vi "Car Wash.vi"() -> ()   [LabVIEW 2018]
uses:
  Controls/Car Wash Indicators.ctl
  Controls/Wash Options.ctl
  Controls/Timer Parameters.ctl
  Controls/FGV Timer Control.ctl
  Controls/UI Data Car Wash.ctl
  Controls/Wash Option Parameters.ctl
  support/Message Queue/Enqueue Message (Single).vi
  <vilib>/Utility/error.llb/Error Cluster From Error Code.vi
  <vilib>/ErrorRing/Error Ring.xnode
  support/Message Queue/Message Queue.lvlib
  support/User Event - Stop/User Event - Stop.lvlib
panel:
  in  "Start":bool
  out "Elapsed Time":dbl format="%0.2f"
  in  "stop":bool
  out "Wash Entry":bool
  in  "Wash Options":T1
  in  "Car Position Slider":u8(slide) max=3 scale=0.0..4.0
  out "Car Wash Indicators":T2
  # "Entry Console"
  # "Car Wash Display"
  # "Car Position Simulation"
  # "Pre-Soak\nH-P Wash\nL-P Wax\nSpot Free Rinse"
  # "Underbody Wash\nBug Remover"
  # "Tire Shine\nAir Dry"
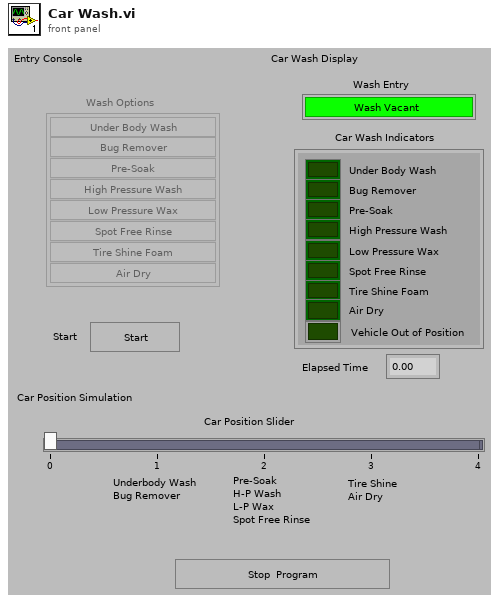
[diagram p1: front panel]
types:
  T1 = typedef "Wash Options.ctl" = cluster{"Underbody Wash":bool, "Bug Remover":bool, "Pre-Soak":bool, "High Pressure Wash":bool, "Low Pressure Wax":bool, "Spot Free Rinse":bool, "Tire Shine Foam":bool, "Air Dry":bool}
  T2 = typedef "Car Wash Indicators.ctl" = cluster{"Under Body Wash":bool, "Bug Remover":bool, "Pre-Soak":bool, "High Pressure Wash":bool, "Low Pressure Wax":bool, "Spot Free Rinse":bool, "Tire Shine Foam":bool, "Air Dry":bool, "Vehicle Out of Position":bool}
  T3 = typedef "UI Data Car Wash.ctl" = cluster{"Underbody Wash Ref":refnum<vi>, "Bug Remover Ref":refnum<vi>, "Pre-Soak Ref":refnum<vi>, "High Pressure Ref":refnum<vi>, "Low Pressure Ref":refnum<vi>, "Spot Free Rinse Ref":refnum<vi>, "Tire Shine Foam Ref":refnum<vi>, "Air Dry Ref":refnum<vi>}
  T4 = typedef "Timer Parameters.ctl" = cluster{"Time Target":dbl, "Timer Mode":T5}
  T5 = typedef "FGV Timer Control.ctl" = enum16{"Start Time", "Read Time", "Pause", "Resume"}
  T6 = typedef "Message Queue.lvlib/All Message Queues.ctl" = cluster{"UI":refnum<queue>}
  T7 = enum8{"Enabled", "Disabled", "Disabled and Grayed Out"}
  T8 = typedef "Wash Option Parameters.ctl" = cluster{"Wash Option":string, "Time":i32, "Station":i32}
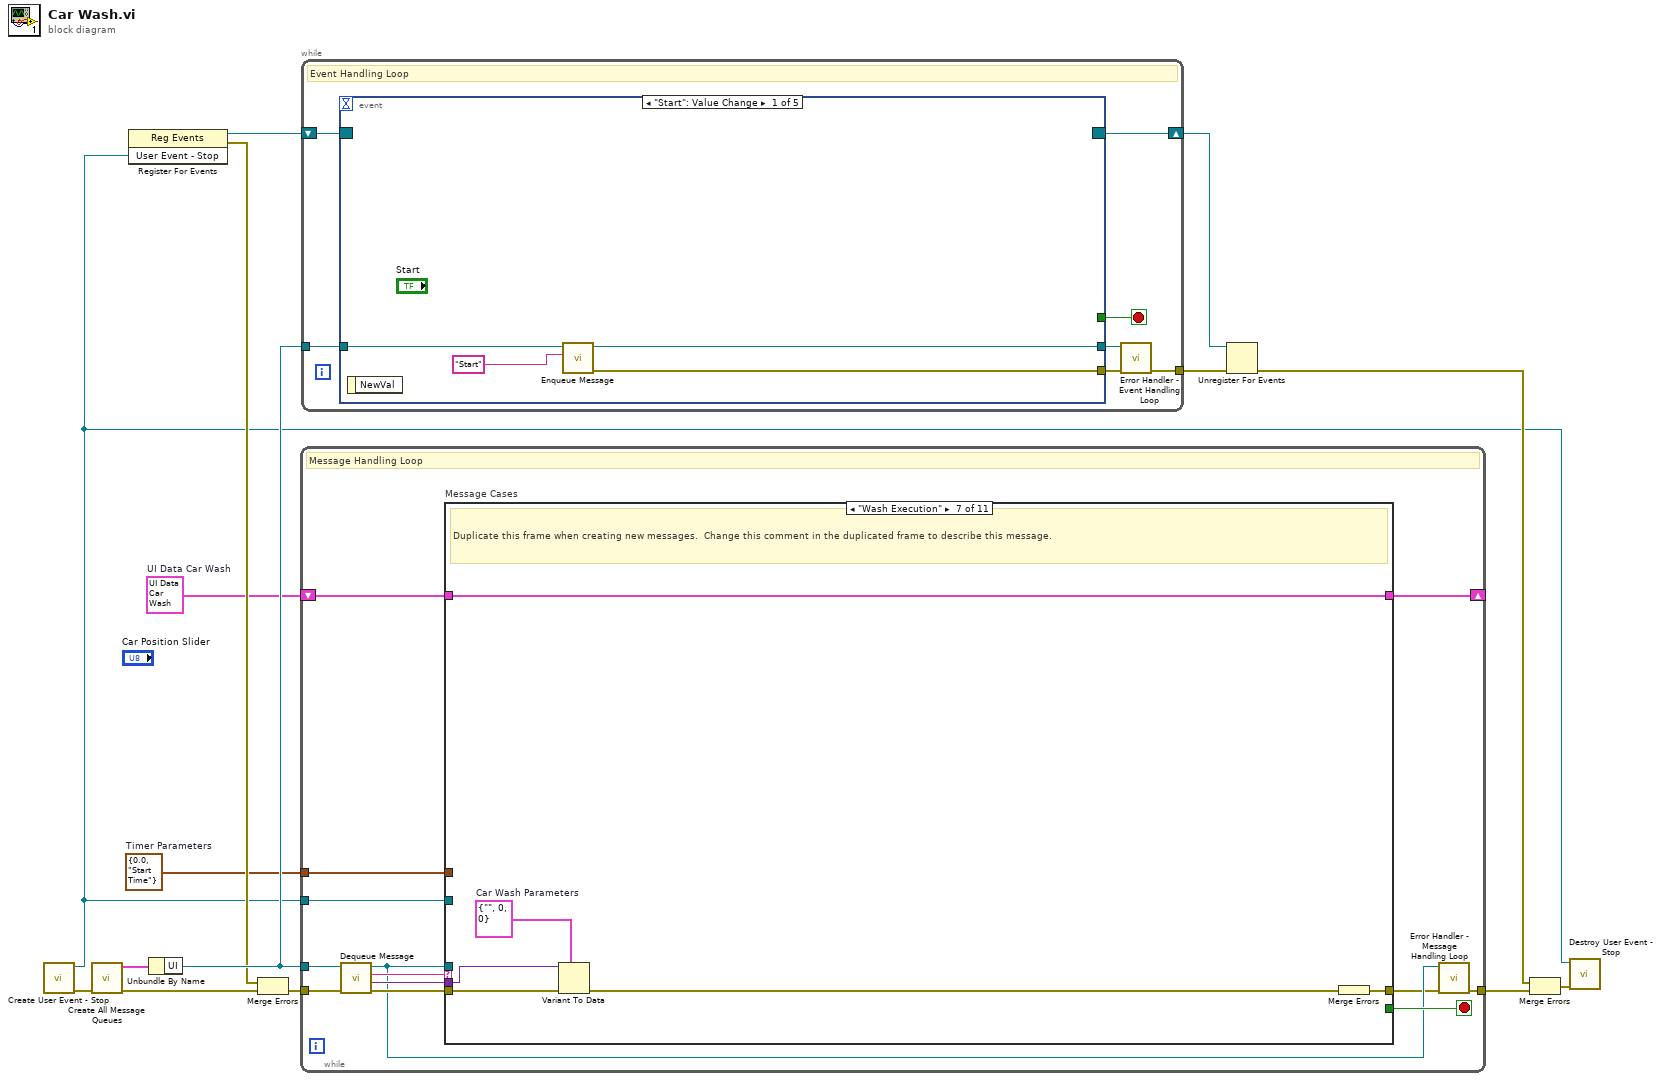
[diagram p0: block diagram]
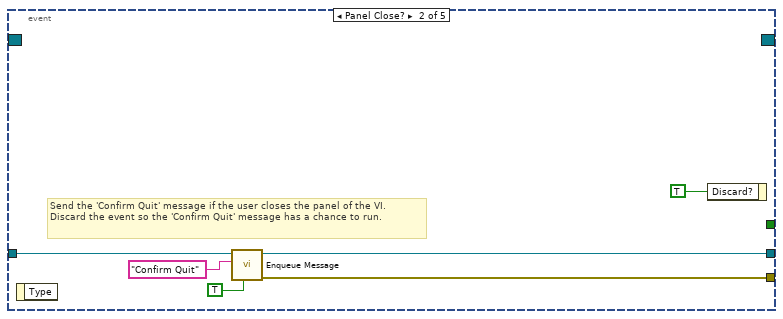
[diagram p2: hidden frame]
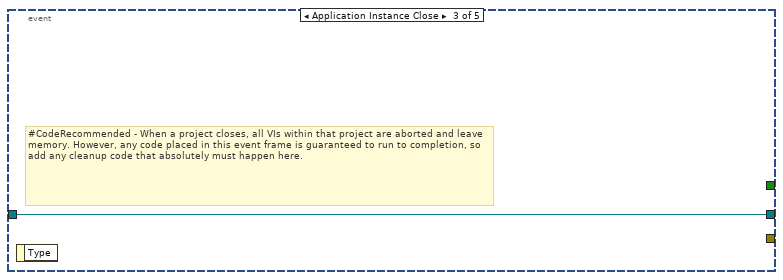
[diagram p3: hidden frame]
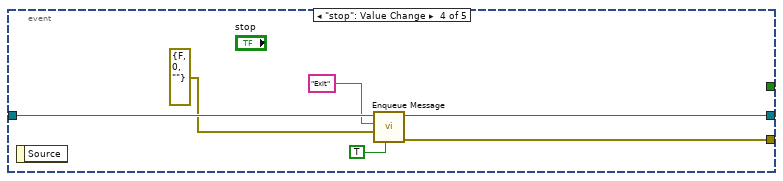
[diagram p4: hidden frame]
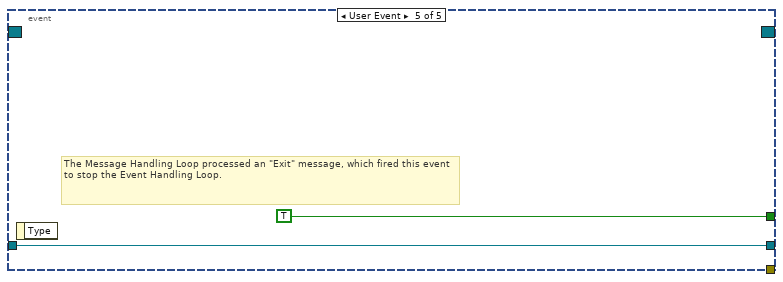
[diagram p5: hidden frame]
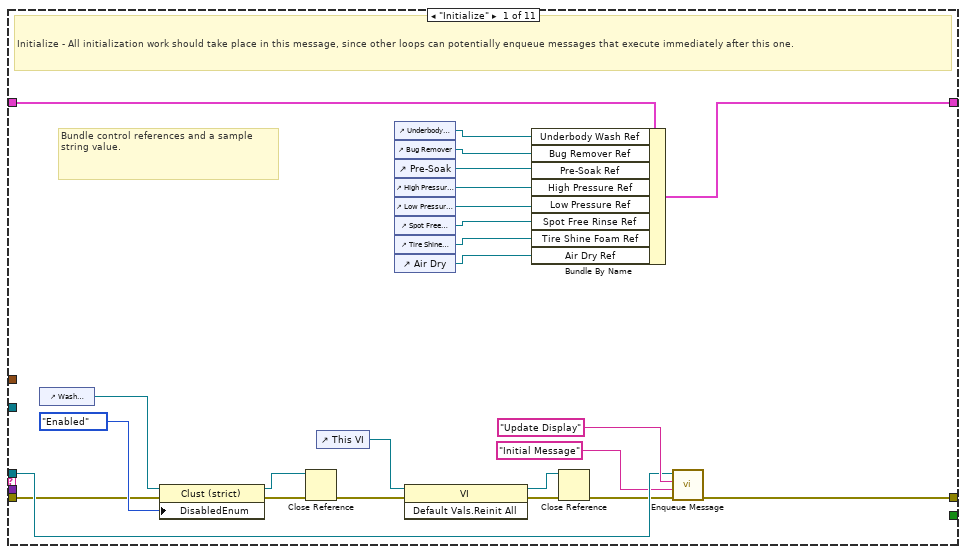
[diagram p6: hidden frame]
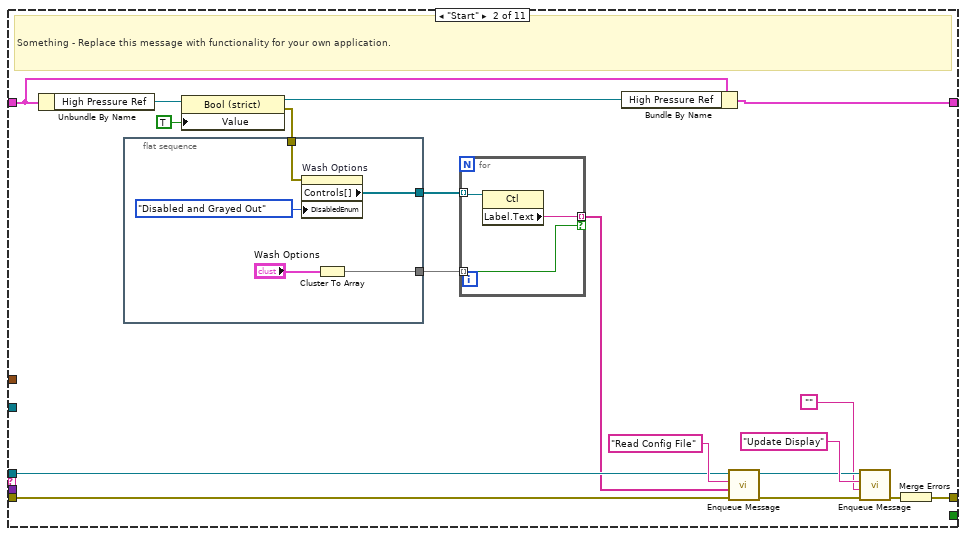
[diagram p7: hidden frame]
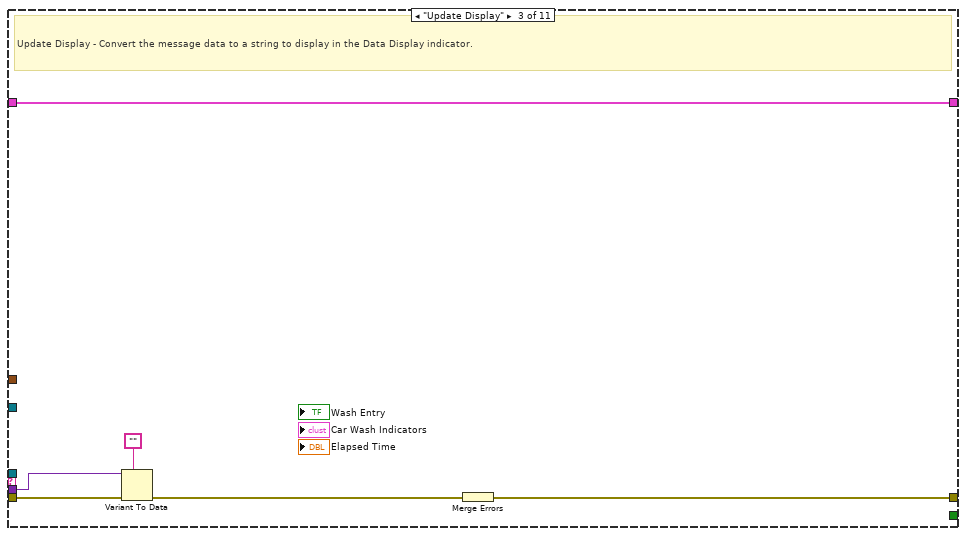
[diagram p8: hidden frame]
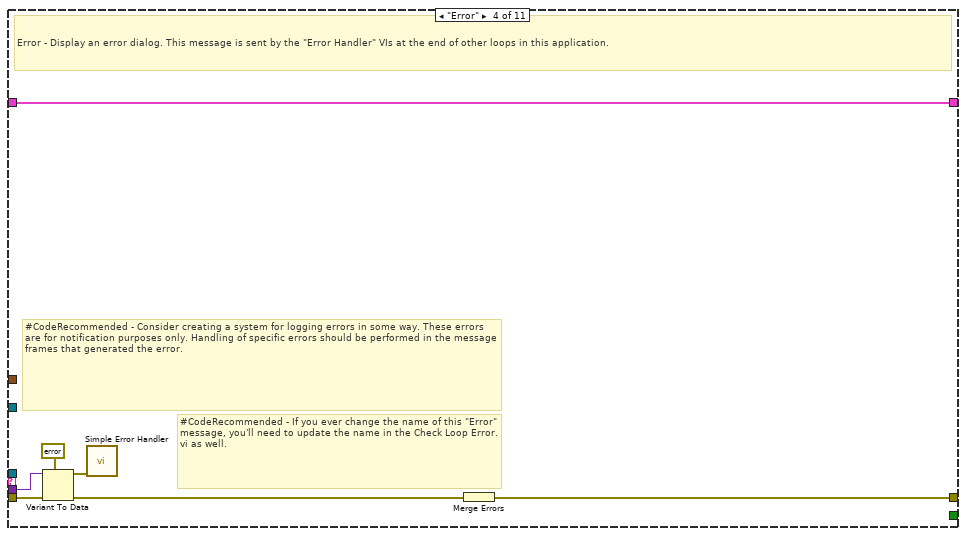
[diagram p9: hidden frame]
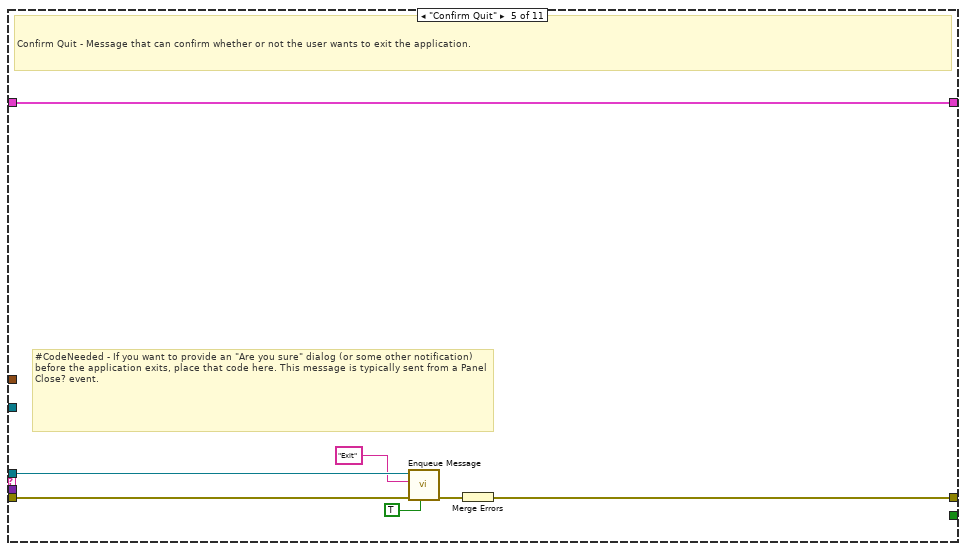
[diagram p10: hidden frame]
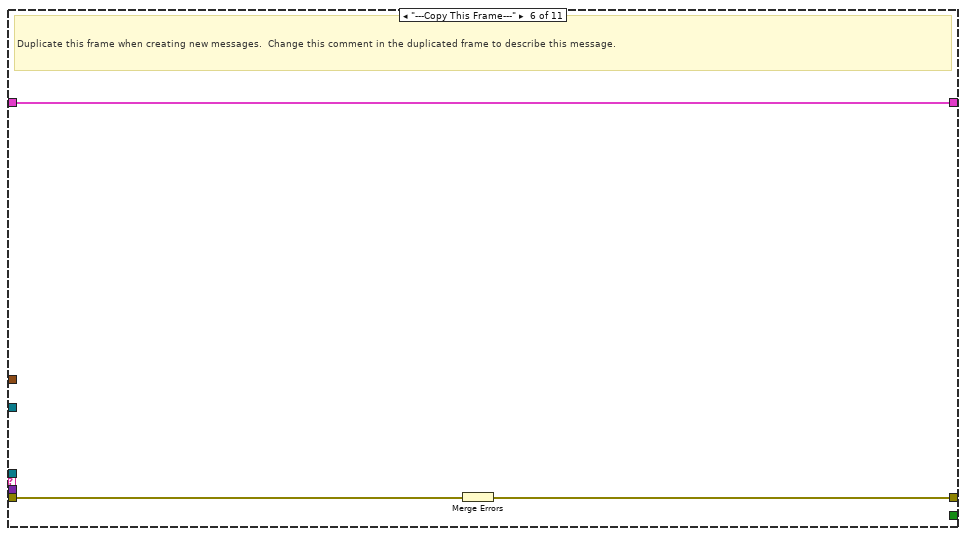
[diagram p11: hidden frame]
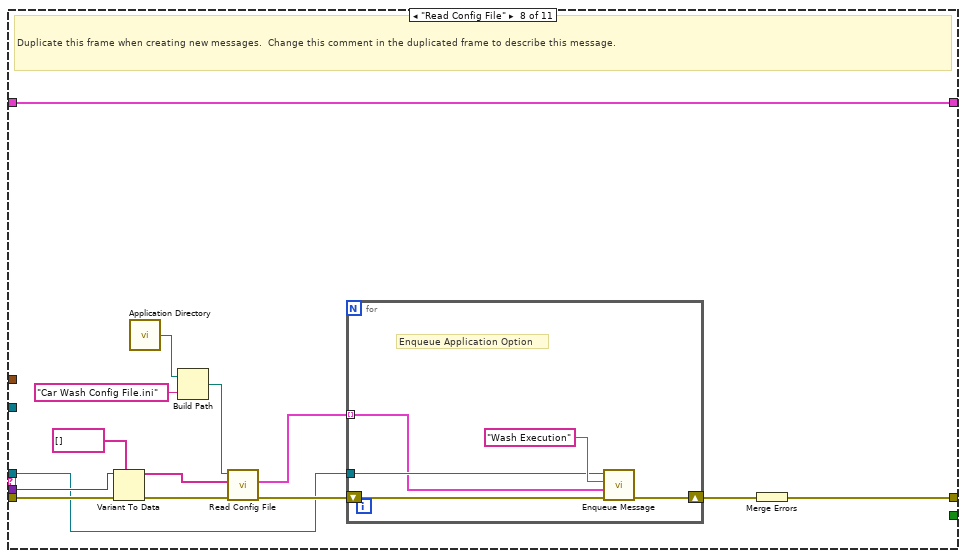
[diagram p12: hidden frame]
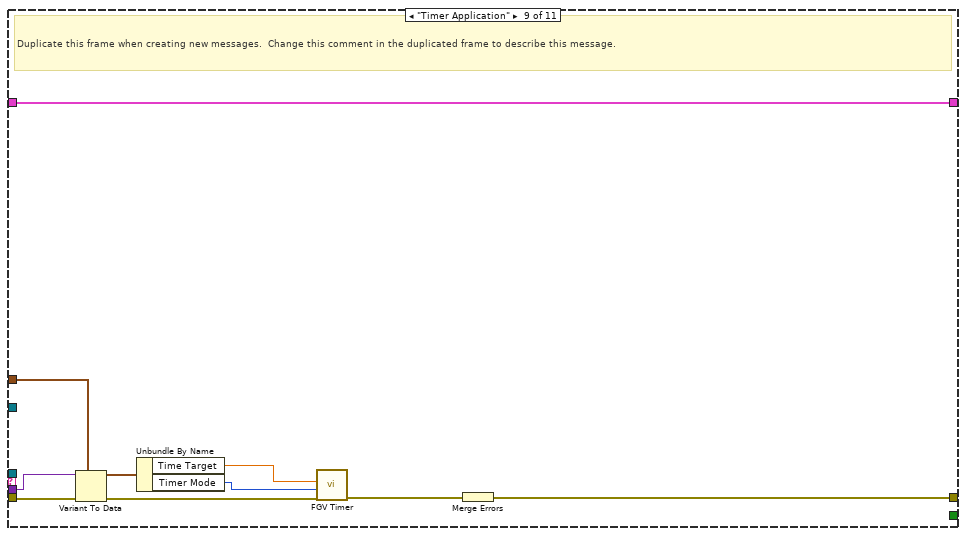
[diagram p13: hidden frame]
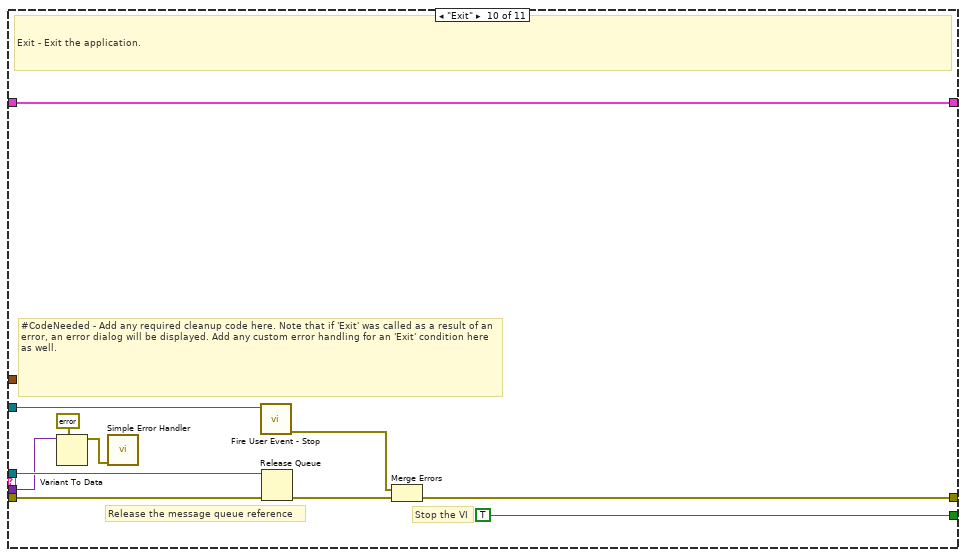
[diagram p14: hidden frame]
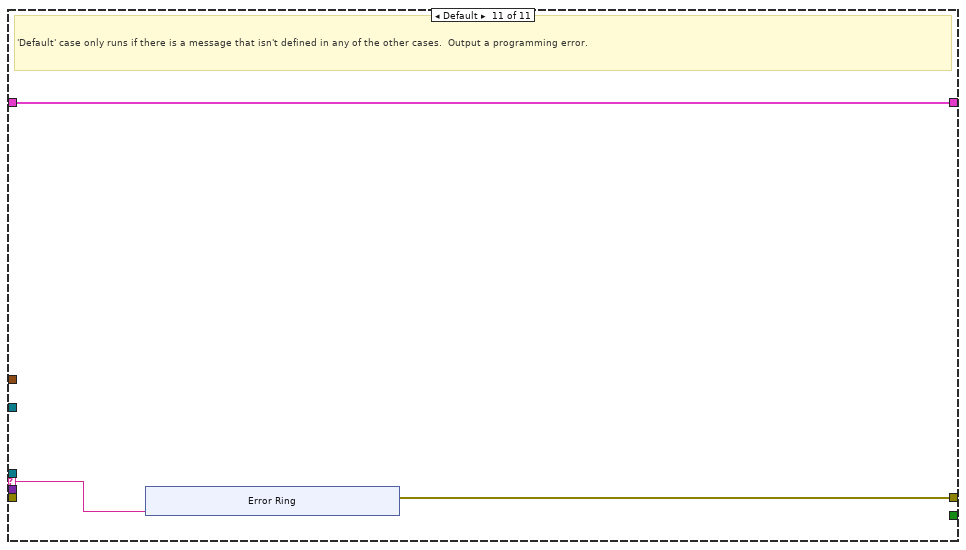
[diagram p15: hidden frame]
diagram:
  w1 = T3 {"Underbody Wash Ref"=refnum, "Bug Remover Ref"=refnum, "Pre-Soak Ref"=refnum, "High Pressure Ref"=refnum, "Low Pressure Ref"=refnum, "Spot Free Rinse Ref"=refnum, "Tire Shine Foam Ref"=refnum, "Air Dry Ref"=refnum}  # UI Data Car Wash
  w2 = T4 {"Time Target"=0.0, "Timer Mode"=enum."Start Time"}  # Timer Parameters
  n1 = call "Create User Event - Stop.vi"() -> ("error out"=w11:errorcluster, "User Event - Stop"=w3:refnum<user-event>)  [unwired: 10 in]
  n2 = call "Create All Message Queues.vi"("error in (no error)"=w11) -> ("error out"=w15:errorcluster, "Message Queues out"=w14:T6)  [unwired: 9 in]
  n3 = register-events(w3) -> (reference out=w6:refnum<event-registration>, error out=w4:errorcluster)  [unwired: 2 in]
  n4 = Unbundle By Name(w14) -> ("UI"=w12:refnum<queue>)
  n5 = Merge Errors(w4, w15) -> (w5:errorcluster)
  n6 = while {
    tunnel: w12 -> [w20]
    shift-right: [w27] -> _
    shift-left: w1 -> [w28]
    tunnel: w3 -> [w25]
    tunnel: w5 -> [w24]
    tunnel: [w18] -> w13
    tunnel: w2 -> [w16]
    stop <- w26 stop-if-true
    # "Message Handling Loop"
    n7 = call "Dequeue Message.vi"("error in (no error)"=w24, "Message Queue"=w20) -> ("error out"=w23:errorcluster, "Message Data"=w21:variant, "Message"=w22:string, "dup Message Queue"=w19:refnum<queue>)  [unwired: 6 in]
    n8 = case "Message Cases" shown="\"Wash Execution\"" w22 {
      selector: w22 -> [_ _ _ _ _ _ _ _ _ _ w148]
      tunnel: w19 -> [w50 w63 _ _ w94 _ _ w110 _ w147 _]
      tunnel: w23 -> [w32 w65 w82 w91 w98 w101 w105 w119 w134 w140 _]
      tunnel: [w52 w70 w83 w85 w96 w99 w106 w120 w136 w143 w149] -> w17
      tunnel: w28 -> [w40 w56 w84 w90 w97 w100 w107 w121 w127 w146 w150]
      tunnel: [w39 w54 w84 w90 w97 w100 w107 w121 w127 w146 w150] -> w27
      tunnel: [_ _ _ _ _ _ _ _ _ TRUE _] -> w26
      tunnel: w21 -> [_ _ w81 w89 _ _ w104 w113 w132 w137 _]
      tunnel: w25 -> [_ _ _ _ _ _ _ _ _ w142 _]
      tunnel: w16 -> [_ _ _ _ _ _ _ _ w131 _ _]
      frame "Initialize" {
        # "Bundle control references and a sample string value."
        # "Initialize - All initialization work should take place in this message, since other loops can potentially enqueue messages that execute immediately after this one."
        n9 = control-ref of="Wash Options"() -> (w34:refnum<vi>)
        n10 = property class="Clust (strict)"(reference=w34, error in=w32, "DisabledEnum"=T7."Enabled" ("Disabled")) -> (reference out=w29:refnum<vi>, error out=w31:errorcluster)
        n11 = Close Reference(reference=w29, error in (no error)=w31) -> (error out=w30:errorcluster)
        n12 = control-ref of="This VI"() -> (w35:refnum<vi>)
        n13 = control-ref of="Underbody Wash"() -> (w43:refnum<vi>)
        n14 = control-ref of="Bug Remover"() -> (w44:refnum<vi>)
        n15 = control-ref of="Pre-Soak"() -> (w45:refnum<vi>)
        n16 = control-ref of="High Pressure Wash"() -> (w48:refnum<vi>)
        n17 = control-ref of="Low Pressure Wax"() -> (w47:refnum<vi>)
        n18 = control-ref of="Spot Free Rinse"() -> (w46:refnum<vi>)
        n19 = control-ref of="Tire Shine Foam"() -> (w42:refnum<vi>)
        n20 = control-ref of="Air Dry"() -> (w41:refnum<vi>)
        n21 = invoke class="VI" method="Default Vals.Reinit All"(reference=w35, error in=w30) -> (reference out=w38:refnum<vi>, error out=w37:errorcluster)  [unwired: 1 in, 1 out]
        n22 = Bundle By Name(cluster=w40, "Underbody Wash Ref"=w43, "Bug Remover Ref"=w44, "Pre-Soak Ref"=w45, "High Pressure Ref"=w48, "Low Pressure Ref"=w47, "Spot Free Rinse Ref"=w46, "Tire Shine Foam Ref"=w42, "Air Dry Ref"=w41) -> (w39:T3)
        n23 = Close Reference(reference=w38, error in (no error)=w37) -> (error out=w36:errorcluster)
        n24 = call-poly "Enqueue Message.vi"("error in (no error)"=w36, "Message Data"="Initial Message" ("Initial Message"), "Message"="Update Display", "Message Queue"=w50) -> ("error out"=w52:errorcluster)  [unwired: 6 in, 1 out]
      }
      frame "Start" {
        # "Something - Replace this message with functionality for your own application."
        n25 = Unbundle By Name(w56) -> ("High Pressure Ref"=w62:refnum<vi>)
        n26 = flat-sequence {
          tunnel: w60 -> [w75]
          tunnel: [w73] -> w59
          tunnel: [w72] -> w58
          frame #0 {
            n27 = property on="Wash Options" class="Clust (strict)"(error in=w75, "DisabledEnum"=T7."Disabled and Grayed Out" ("Disabled")) -> ("Controls[]"=w72:refnum<vi>[])  [unwired: 1 in, 2 out]
            n28 = Cluster To Array(cluster="Wash Options") -> (array=w73:bool[])
          }
        }
        n29 = property class="Bool (strict)"(reference=w62, "Value"=TRUE) -> (reference out=w55:refnum<vi>, error out=w60:errorcluster)  [unwired: 1 in]
        n30 = for {
          tunnel: w59 -> [w77] mode=indexing
          tunnel: w58 -> [w78] mode=indexing
          tunnel: [w76] -> w57 mode=indexing if=w77
          n31 = property class="Ctl"(reference=w78) -> ("Label.Text"=w76:string)  [unwired: 1 in, 2 out]
        }
        n32 = Bundle By Name(cluster=w56, "High Pressure Ref"=w55) -> (w54:T3)
        n33 = call-poly "Enqueue Message.vi"("error in (no error)"=w65, "Message Data"=w57, "Message"="Read Config File", "Message Queue"=w63) -> ("error out"=w66:errorcluster, "dup Message Queue"=w64:refnum<queue>)  [unwired: 6 in]
        n34 = call-poly "Enqueue Message.vi"("error in (no error)"=w66, "Message Data"="", "Message"="Update Display", "Message Queue"=w64) -> ("error out"=w69:errorcluster)  [unwired: 6 in, 1 out]
        n35 = Merge Errors(w69) -> (w70:errorcluster)
      }
      frame "Update Display" {
        # "Update Display - Convert the message data to a string to display in the Data Display indicator."
        n36 = Variant To Data(error in=w82, type="", Variant=w81) -> (error out=w79:errorcluster)  [unwired: 1 out]
        n37 = Merge Errors(w79) -> (w83:errorcluster)
      }
      frame "Error" {
        # "#CodeRecommended - If you ever change the name of this \"Error\" message, you'll need to update the name in the Check Loop Error.vi as well."
        # "#CodeRecommended - Consider creating a system for logging errors in some way. These errors are for notification purposes only. Handling of specific errors should be performed in the message frames that generated the error."
        # "Error - Display an error dialog. This message is sent by the \"Error Handler\" VIs at the end of other loops in this application."
        n38 = Variant To Data(error in=w91, type=errorcluster {"status"=FALSE, "code"=0, "source"=""} ("error constant"), Variant=w89) -> (data=w87:errorcluster, error out=w86:errorcluster)
        n39 = call <vilib>:"Simple Error Handler.vi"("error in (no error)"=w87) -> ()  [unwired: 4 in, 5 out]
        n40 = Merge Errors(w86) -> (w85:errorcluster)
      }
      frame "Confirm Quit" {
        # "#CodeNeeded - If you want to provide an \"Are you sure\" dialog (or some other notification) before the application exits, place that code here. This message is typically sent from a Panel Close? event."
        # "Confirm Quit - Message that can confirm whether or not the user wants to exit the application."
        n41 = call-poly "Enqueue Message.vi"("Priority Message? (F)"=TRUE, "error in (no error)"=w98, "Message"="Exit", "Message Queue"=w94) -> ("error out"=w95:errorcluster)  [unwired: 6 in, 1 out]
        n42 = Merge Errors(w95) -> (w96:errorcluster)
      }
      frame "---Copy This Frame---" {
        # "Duplicate this frame when creating new messages.  Change this comment in the duplicated frame to describe this message."
        n43 = Merge Errors(w101) -> (w99:errorcluster)
      }
      frame "Wash Execution" {
        w103 = T8 {"Wash Option"="", "Time"=0, "Station"=0}  # Car Wash Parameters
        # "Duplicate this frame when creating new messages.  Change this comment in the duplicated frame to describe this message."
        n44 = Variant To Data(error in=w105, type=w103, Variant=w104) -> (error out=w102:errorcluster)  [unwired: 1 out]
        n45 = Merge Errors(w102) -> (w106:errorcluster)
      }
      frame "Read Config File" {
        # "Duplicate this frame when creating new messages.  Change this comment in the duplicated frame to describe this message."
        n46 = Variant To Data(error in=w119, type=string[] [], Variant=w113) -> (data=w114:string[], error out=w118:errorcluster)
        n47 = call <vilib>:"Application Directory.vi"() -> ("Application Directory"=w117:path)
        n48 = Build Path(base path=w117, name or relative path="Car Wash Config File.ini") -> (appended path=w116:path)
        n49 = call "Read Config File.vi"("Error In"=w118, "Wash Options"=w114, "File Path Control"=w116) -> ("Error Out"=w111:errorcluster, "Wash Option Parameters"=w108:T8[])  [unwired: 7 in]
        n50 = for {
          tunnel: w110 -> [w124]
          shift-right: [w123] -> w109
          shift-left: w111 -> [w125]
          tunnel: w108 -> [w122] mode=indexing
          # "Enqueue Application Option"
          n51 = call-poly "Enqueue Message.vi"("error in (no error)"=w125, "Message Data"=w122, "Message"="Wash Execution", "Message Queue"=w124) -> ("error out"=w123:errorcluster)  [unwired: 6 in, 1 out]
        }
        n52 = Merge Errors(w109) -> (w120:errorcluster)
      }
      frame "Timer Application" {
        # "Duplicate this frame when creating new messages.  Change this comment in the duplicated frame to describe this message."
        n53 = Variant To Data(error in=w134, type=w131, Variant=w132) -> (data=w130:T4, error out=w133:errorcluster)
        n54 = Unbundle By Name(w130) -> ("Time Target"=w128:dbl, "Timer Mode"=w129:T5)
        n55 = call "FGV Timer.vi"("Error In"=w133, "Timer Mode"=w129, "Time Target (s)"=w128) -> ("Error Out"=w135:errorcluster)  [unwired: 6 in, 2 out]
        n56 = Merge Errors(w135) -> (w136:errorcluster)
      }
      frame "Exit" {
        # "Stop the VI"
        # "Release the message queue reference"
        # "#CodeNeeded - Add any required cleanup code here. Note that if 'Exit' was called as a result of an error, an error dialog will be displayed. Add any custom error handling for an 'Exit' condition here as well."
        # "Exit - Exit the application."
        n57 = Variant To Data(type=errorcluster {"status"=FALSE, "code"=0, "source"=""} ("error constant"), Variant=w137) -> (data=w138:errorcluster)  [unwired: 1 in, 1 out]
        n58 = call <vilib>:"Simple Error Handler.vi"("error in (no error)"=w138) -> ()  [unwired: 4 in, 5 out]
        n59 = call "Fire User Event - Stop.vi"("User Event - Stop"=w142) -> ("error out"=w141:errorcluster)  [unwired: 10 in]
        n60 = Release Queue(queue=w147, error in (no error)=w140) -> (error out=w144:errorcluster)  [unwired: 1 in, 2 out]
        n61 = Merge Errors(w141, w144) -> (w143:errorcluster)
      }
      frame Default {
        # "'Default' case only runs if there is a message that isn't defined in any of the other cases.  Output a programming error."
        n62 = xnode "Error Ring"("parameter 0"=w148) -> ("error out"=w149:errorcluster)
      }
    }
    n63 = call "Error Handler - Message Handling Loop.vi"("error in (no error)"=w17, "Message Queue"=w19) -> ("dup error in"=w18:errorcluster)  [unwired: 8 in, 1 out]
  }
  n64 = while {
    tunnel: w12 -> [w164]
    shift-right: [w162] -> w8
    shift-left: w6 -> [w163]
    tunnel: [w158] -> w7
    stop <- w160 stop-if-true
    # "Event Handling Loop"
    n65 = event shown="[0] \"Start\": Value Change" {
      selector: w163 -> [_ _ _ _ _]
      dyn-events: [_ _ _ _ _] -> w162
      timeout: _ -> [_ _ _ _ _]
      tunnel: [_ _ _ _ TRUE ("Discard?")] -> w160
      tunnel: w164 -> [w168 w173 w175 w181 w183]
      tunnel: [w165 w172 _ w180 _] -> w161
      tunnel: [w167 w171 w175 w179 w183] -> w159
      event "Start": Value Change {
        n66 = event-data() -> ()  [unwired: 1 in, 1 out]
        n67 = call-poly "Enqueue Message.vi"("Message"="Start", "Message Queue"=w168) -> ("error out"=w165:errorcluster, "dup Message Queue"=w167:refnum<queue>)  [unwired: 8 in]
      }
      event Panel Close? {
        # "Send the 'Confirm Quit' message if the user closes the panel of the VI. Discard the event so the 'Confirm Quit' message has a chance to run."
        n68 = event-data() -> ()  [unwired: 1 in, 1 out]
        n69 = call-poly "Enqueue Message.vi"("Priority Message? (F)"=TRUE, "Message"="Confirm Quit", "Message Queue"=w173) -> ("error out"=w172:errorcluster, "dup Message Queue"=w171:refnum<queue>)  [unwired: 7 in]
        n70 = event-data("Discard?"=TRUE) -> ()  [unwired: 1 in, 1 out]
      }
      event Application Instance Close {
        # "#CodeRecommended - When a project closes, all VIs within that project are aborted and leave memory. However, any code placed in this event frame is guaranteed to run to completion, so add any cleanup code that absolutely must happen here."
        n71 = event-data() -> ()  [unwired: 1 in, 1 out]
      }
      event "stop": Value Change {
        n72 = event-data() -> ()  [unwired: 1 in, 1 out]
        n73 = call-poly "Enqueue Message.vi"("Priority Message? (F)"=TRUE, "Message Data"=errorcluster {"status"=FALSE, "code"=0, "source"=""} ("error out"), "Message"="Exit", "Message Queue"=w181) -> ("error out"=w180:errorcluster, "dup Message Queue"=w179:refnum<queue>)  [unwired: 6 in]
      }
      event User Event {
        # "The Message Handling Loop processed an \"Exit\" message, which fired this event to stop the Event Handling Loop."
        n74 = event-data() -> ()  [unwired: 1 in, 1 out]
      }
    }
    n75 = call "Error Handler - Event Handling Loop.vi"("error in (no error)"=w161, "Message Queue"=w159) -> ("dup error in"=w158:errorcluster)  [unwired: 8 in, 1 out]
  }
  n76 = Unregister For Events(event registration refnum=w8, error in=w7) -> (error out=w9:errorcluster)
  n77 = Merge Errors(w9, w13) -> (w10:errorcluster)
  n78 = call "Destroy User Event - Stop.vi"("error in (no error)"=w10, "User Event - Stop"=w3) -> ()  [unwired: 9 in, 1 out]
